vi "time_array_test.vi"() -> ()   [LabVIEW 2017]
panel:
  out "Array":dbl[][](array[numeric])
  out "appended array":dbl[][][](array[numeric])
  out "最近五筆大於0.9":dbl[][](array[numeric])
  out "最近五筆小於0.9":dbl[][](array[numeric])
  out "最新十筆":dbl[][](array[numeric])
  out "控制指示燈":bool
  in  "迴圈速率":u32
  out "最新數據":dbl[](array[numeric])
  out "day":dbl(knob) scale=0.0..10.0
  out "hr":dbl(knob) scale=0.0..10.0
  out "min":dbl(knob) scale=0.0..60.0
  out "迴圈次數":i32
  in  "stop":bool
  out "s":dbl(knob) scale=0.0..60.0
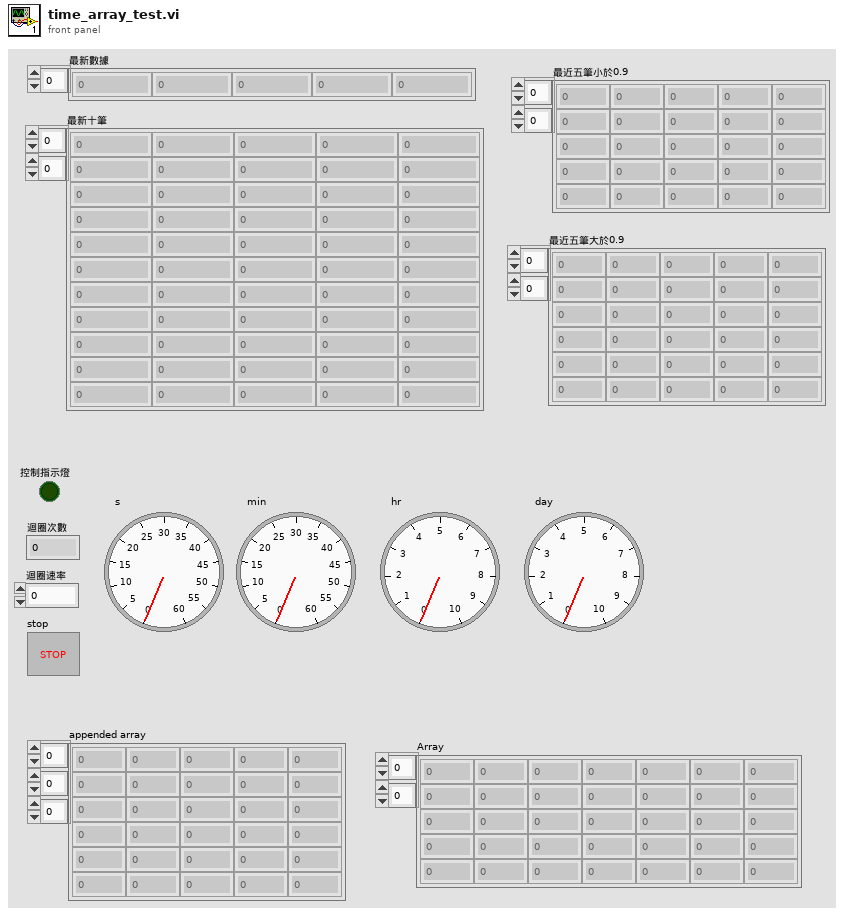
[diagram p1: front panel]
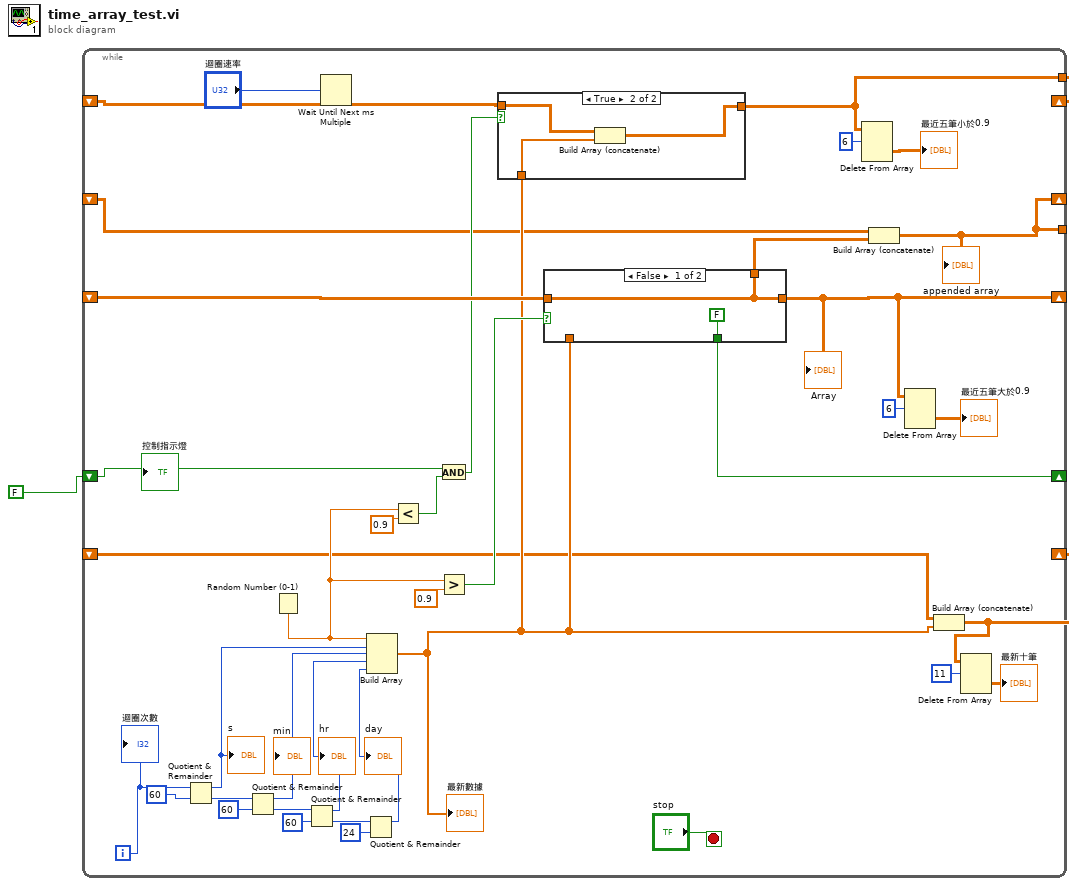
[diagram p0: block diagram]
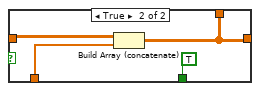
[diagram p3: hidden frame]
diagram:
  n1 = while {
    shift-right: [w5] -> _
    shift-left: _ -> [w24]
    shift-right: [w23] -> _
    shift-left: FALSE -> [w19]
    shift-right: [w2] -> _
    shift-left: _ -> [w16]
    shift-right: [w11] -> _
    shift-left: _ -> [w12]
    shift-right: [w3] -> _
    shift-left: _ -> [w6]
    tunnel: [w3] -> _
    tunnel: [w2] -> _
    i -> [w38]
    stop <- "stop" stop-if-true
    n2 = Quotient & Remainder(x=w38, y=60) -> (x-y*floor(x/y)=w30:i32, floor(x/y)=w36:i32)
    "s" <- w30
    n3 = Quotient & Remainder(x=w36, y=60) -> (x-y*floor(x/y)=w29:i32, floor(x/y)=w34:i32)
    "min" <- w29
    n4 = Random Number (0-1)() -> (number: 0 to 1=w20:dbl)
    n5 = Quotient & Remainder(x=w34, y=60) -> (x-y*floor(x/y)=w28:i32, floor(x/y)=w32:i32)
    "hr" <- w28
    n6 = Wait Until Next ms Multiple(millisecond multiple="迴圈速率") -> ()  [unwired: 1 out]
    n7 = Quotient & Remainder(x=w32, y=24) -> (x-y*floor(x/y)=w27:i32)  [unwired: 1 out]
    "day" <- w27
    n8 = Build Array(w20, w30, w29, w28, w27) -> (w13:dbl[])
    "最新數據" <- w13
    n9 = Less?(x=w20, y=0.9) -> (x < y?=w18:bool)
    n10 = And(x=w19, y=w18) -> (x .and. y?=w17:bool)
    n11 = Greater?(x=w20, y=0.9) -> (0:w22:bool)
    n12 = case shown="True" w17 {
      tunnel: w16 -> [w40 w43]
      tunnel: [w40 w41] -> w2
      tunnel: w13 -> [_ w42]
      frame False {
      }
      frame True {
        n13 = Build Array (concatenate)(w43, w42) -> (w41:dbl[][])
      }
    }
    n14 = case shown="False" w22 {
      tunnel: w13 -> [_ w47]
      tunnel: w24 -> [w44 w49]
      tunnel: [w44 w46] -> w5
      tunnel: [FALSE TRUE] -> w23
      tunnel: [w44 w46] -> w4
      frame False {
      }
      frame True {
        n15 = Build Array (concatenate)(w49, w47) -> (w46:dbl[][])
      }
    }
    "Array" <- w5
    n16 = Delete From Array(array=w2, length=6) -> (deleted portion=→"最近五筆小於0.9":dbl[][])  [unwired: 2 in, 1 out]
    n17 = Build Array (concatenate)(w6, w4) -> (w3:dbl[][][])
    "appended array" <- w3
    n18 = Delete From Array(array=w5, length=6) -> (deleted portion=→"最近五筆大於0.9":dbl[][])  [unwired: 2 in, 1 out]
    n19 = Build Array (concatenate)(w12, w13) -> (w11:dbl[][])
    n20 = Delete From Array(array=w11, length=11) -> (deleted portion=→"最新十筆":dbl[][])  [unwired: 2 in, 1 out]
    "迴圈次數" <- w38
    "控制指示燈" <- w19
  }
